vi "Utils - SetImageProperties.vi"(8 "error in (no error)":errorcluster, 11 "xiCam In":refnum<k24>) -> (0 "error out":errorcluster, 3 "xiCam Out":refnum<k24>)   [LabVIEW 2016]
doc: "Low level VI. xiApi calls this VI when image size has changed for example: Downsampling mode or Set Image Width and Height."
uses:
  C:/Users/Ries Lab/Documents/Microscope Control from Sheng Account/Microscope-Control/Device Library/Cameras/Ximea/xiLIB_64bit/xiLIB/xiCamLib/API/x64/xiApi.NETX64.dll
  API/x64/xiApi.NETX64.dll
  xiImageManager/xiImageMng - State.ctl
  PRM/IMG_FORMAT/IMG_DATA_FORMAT.ctl
  PRM/PRM/PRM_v2.ctl
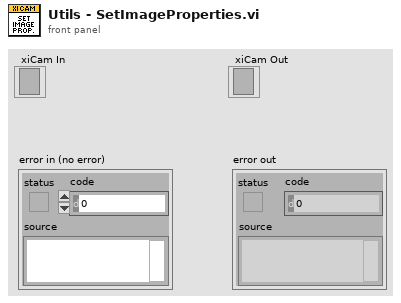
[diagram p1: front panel]
types:
  T1 = typedef "PRM_v2.ctl" = enum16{"ACQ_BUFFER_SIZE", "ACQ_FRAME_BURST_COUNT", "ACQ_TIMING_MODE", "ACQ_TRANSPORT_BUFFER_SIZE", "AE_MAX_LIMIT", "AEAG", "AEAG_LEVEL", "API_VERSION", "AG_MAX_LIMIT", "APPLY_CMS", "AUTO_BANDWIDTH_CALCULATION", "AUTO_WB", "AVAILABLE_BANDWIDTH", "AVAILABLE_BANDWIDTH_MAX", "AVAILABLE_BANDWIDTH_MIN", "BUFFER_POLICY", "BUFFERS_QUEUE_SIZE", "CC_MATRIX_00", "CC_MATRIX_01", "CC_MATRIX_02", "CC_MATRIX_03", "CC_MATRIX_10", "CC_MATRIX_11", "CC_MATRIX_12", "CC_MATRIX_13", "CC_MATRIX_20", "CC_MATRIX_21", "CC_MATRIX_22", "CC_MATRIX_23", "CC_MATRIX_30", "CC_MATRIX_31", "CC_MATRIX_32", "CC_MATRIX_33", "CHIP_TEMP", "CMS", "COLOR_FILTER_ARRAY", "COOLING", "DEBOUNCE_EN", "DEBOUNCE_POL", "DEBOUNCE_T0", "DEBOUNCE_T1", "DEBUG_LEVEL", "DEFAULT_CC_MATRIX", "DEVICE_INSTANCE_PATH", "DEVICE_MODEL_ID", "DEVICE_NAME", "DEVICE_SN", "DEVICE_TYPE", "DEVICE_USER_ID", "DOWNSAMPLING", "DOWNSAMPLING_TYPE", "DRV_VERSION", "EXP_PRIORITY", "EXPOSURE", "EXPOSURE_MAX", "EXPOSURE_MIN", "FFS_FILE_NAME", "FPGA1_VERSION", "FRAMERATE", "FRAMERATE_MAX", "FRAMERATE_MIN", "FREE_FFS_SIZE", "GAIN", "GAIN_MAX", "GAIN_MIN", "GAMMAC", "GAMMAY", "GPI_LEVEL", "GPI_MODE", "GPI_SELECTOR", "GPO_MODE", "GPO_SELECTOR", "HDR", "HDR_T1", "HDR_T2", "HEIGHT", "HEIGHT_MAX", "HEIGHT_MIN", "HOUSE_TEMP", "IMAGE_DATA_FORMAT", "IMAGE_IS_COLOR", "INPUT_CMS_PROFILE", "IS_COOLED", "IS_DEVICE_EXIST", "KNEEPOINT1", "KNEEPOINT2", "LED_MODE", "LED_SELECTOR", "LIMIT_BANDWIDTH", "LIMIT_BANDWIDTH_MAX", "LIMIT_BANDWIDTH_MIN", "LUT_EN", "LUT_INDEX", "LUT_INDEX_MAX", "LUT_INDEX_MIN", "LUT_VALUE", "LUT_VALUE_MAX", "LUT_VALUE_MIN", "MANUAL_WB", "MCU1_VERSION", "MCU2_VERSION", "OFFSET_X", "OFFSET_X_MAX", "OFFSET_X_MIN", "OFFSET_Y", "OFFSET_Y_MAX", "OFFSET_Y_MIN", "OUTPUT_CMS_PROFILE", "OUTPUT_DATA_BIT_DEPTH", "OUTPUT_DATA_PACKING", "READ_FILE_FFS", "RECENT_FRAME", "SENSOR_DATA_BIT_DEPTH", "SENSOR_MODE", "SENSOR_TAPS", "SHARPNESS", "SHUTTER_TYPE", "TARGET_TEMP", "TRG_DELAY", "TRG_SELECTOR", "TRG_SOFTWARE", "TRG_SOURCE", "USED_FFS_SIZE", "WB_KB", "WB_KG", "WB_KR", "WIDTH", "WIDTH_MAX", "WIDTH_MIN", "WRITE_FILE_FFS", "ACQ_BUFFER_SIZE_UNIT", "ACQ_TRANSPORT_BUFFER_COMMIT", "AEAG_ROI_HEIGHT", "AEAG_ROI_OFFSET_X", "AEAG_ROU_OFFSET_Y", "AEAG_ROI_WIDTH", "API_CONTEXT_LIST", "BINNING_HORIZONTAL", "BINNING_SELECTOR", "BINNING_VERTICAL", "COLUMN_FPN_CORRECTION", "COUNTER_SELECTOR", "COUNTER_VALUE", "DECIMATION_HORIZONTAL", "DECIMATION_SELECTOR", "DECIMATION_VERTICAL", "DEVICE_ID", "DEVICE_LOCATION_PATH", "DEVICE_MANIFEST", "DEVICE_RESET", "DEVICE_SENS_SN", "EXPOSURE_BURST_COUNT", "FFS_ACCESS_KEY", "GAIN_SELECTOR", "HW_REVISION", "IMAGE_BLACK_LEVEL", "IMAGE_DATA_BIT_DEPTH", "IMAGE_DATA_FORMAT_RGB32_ALPHA", "IMAGE_PAYLOAD_SIZE", "LENS_APERTURE_VALUE", "LENS_FEATURE", "LENS_FEATURE_SELECTOR", "LENS_FOCAL_LENGTH", "LENS_FOCUS_DISTANCE", "LENS_FOCUS_MOVE", "LENS_FOCUS_MOVEMENT_VALUE", "LENS_MODE", "OUTPUT_DATA_PACKING_TYPE", "SENSOR_CLOCK_FREQ_HZ", "SENSOR_CLOCK_FREQ_INDEX", "SENSOR_FEATURE_SELECTOR", "SENSOR_FEATURE_VALUE", "SENSOR_OUTPUT_CHANNEL_COUNT", "TRANSPORT_PIXEL_FORMAT", "TS_RST_MODE", "TS_RST_SOURCE", "SENS_DEFECTS_CORR_LIST_SELECTOR", "SENS_DEFECTS_CORR", "SENS_DEFECTS_CORR_LIST_CONTENT", "DEVICE_UNIT_SELECTOR", "DEVICE_UNIT_REGISTER_SELECTOR", "DEVICE_UNIT_REGISTER_VALUE"}
  T2 = typedef "IMG_DATA_FORMAT.ctl" = enum16{"MONO8", "MONO16", "RGB24", "RGB32", "RGBPLANAR", "RAW8", "RAW16"}
  T3 = typedef "xiImageMng - State.ctl" = enum16{"Init", "GetProperties", "SetProperties"}
  T4 = cluster{"Int32_Value":i32, "Int32_Value":i32, "IMG_FORMAT":T2}
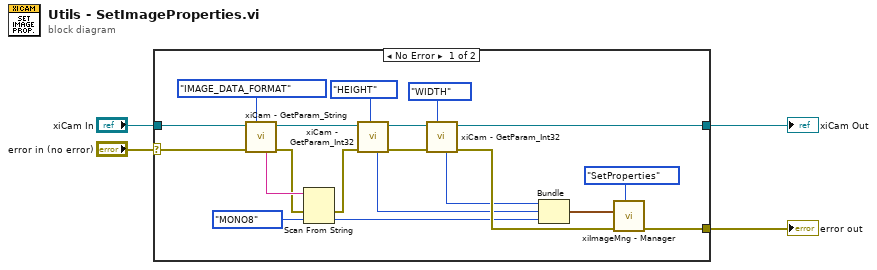
[diagram p0: block diagram]
diagram:
  n1 = case shown="No Error" "error in (no error)" {
    selector: "error in (no error)" -> [w14 w25]
    tunnel: "xiCam In" -> [w15 w26]
    tunnel: [w17 w26] -> w2
    tunnel: [w16 w25] -> w1
    frame No Error {
      n2 = call "xiCam - GetParam_String.vi"("PRM"=PRM_v2."IMAGE_DATA_FORMAT", "error in (no error)"=w14, "xiCam In"=w15) -> ("error out"=w10:errorcluster, "xiCam Out"=w13:refnum<k24>, "String_Value"=w12:string)  [unwired: 6 in]
      n3 = Scan From String(input string=w12, error in=w10, default 1=IMG_DATA_FORMAT."MONO8" ("IMG_FORMAT")) -> (error out=w9:errorcluster, output 1=w8:T2)  [unwired: 2 in, 2 out]
      n4 = call "xiCam - GetParam_Int32.vi"("PRM"=PRM_v2."HEIGHT", "error in (no error)"=w9, "xiCam In"=w13) -> ("error out"=w23:errorcluster, "xiCam Out"=w24:refnum<k24>, "Int32_Value"=w19:i32)  [unwired: 6 in]
      n5 = call "xiCam - GetParam_Int32.vi"("PRM"=PRM_v2."WIDTH", "error in (no error)"=w23, "xiCam In"=w24) -> ("error out"=w21:errorcluster, "xiCam Out"=w17:refnum<k24>, "Int32_Value"=w20:i32)  [unwired: 6 in]
      n6 = Bundle("Int32_Value"=w20, "Int32_Value"=w19, "IMG_FORMAT"=w8) -> (w18:T4)  [unwired: 1 in]
      n7 = call "xiImageMng - Manager.vi"("State"=xiImageMng_-_State."SetProperties", "error in (no error)"=w21, "Properties In"=w18) -> ("error out"=w16:errorcluster)  [unwired: 7 in, 1 out]
    }
    frame Error {
    }
  }
  "error out" <- w1
  "xiCam Out" <- w2
